vi "Write Init.vi"(8 "error in (no error)":errorcluster, 10 "Init":bool, 11 "Mass Flow Controller in":refnum<class "Mass Flow Controller.lvclass">) -> (0 "error out":errorcluster, 3 "Mass Flow Controller out":refnum<class "Mass Flow Controller.lvclass">)   [LabVIEW 2011, in "Mass Flow Controller.lvclass"]
uses:
  Mass Flow Controller.lvclass
  Mass Flow Controller.lvclass/Mass Flow Controller.ctl
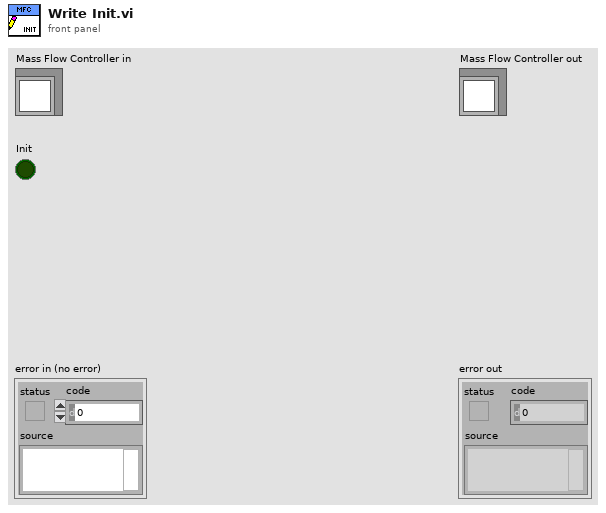
[diagram p1: front panel]
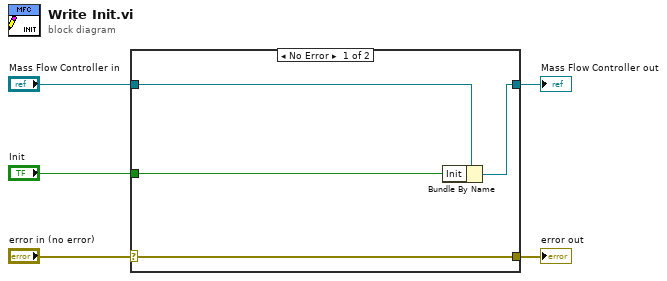
[diagram p0: block diagram]
diagram:
  n1 = case shown="No Error" "error in (no error)" {
    selector: "error in (no error)" -> [w9 w10]
    tunnel: [w9 w10] -> w4
    tunnel: [w7 w11] -> w2
    tunnel: "Mass Flow Controller in" -> [w8 w11]
    tunnel: "Init" -> [w6 _]
    frame No Error {
      n2 = Bundle By Name(cluster=w8, "Init"=w6) -> (w7:refnum<class "Mass Flow Controller.lvclass">)
    }
    frame Error {
    }
  }
  "error out" <- w4
  "Mass Flow Controller out" <- w2
